vi "GUI_ENABLE_ctr (SubVI).vi"(8 "error out 2":errorcluster, 10 "Array":refnum<vi>[](array[refnum]), 11 "Visible":bool) -> (0 "error out":errorcluster)   [LabVIEW 2017]
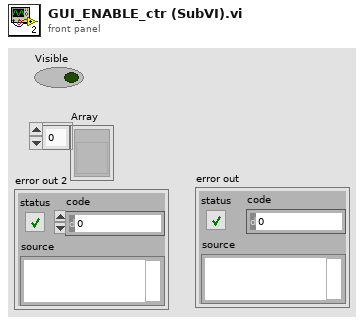
[diagram p1: front panel]
types:
  T1 = enum8{"Enabled", "Disabled", "Disabled and Grayed Out"}
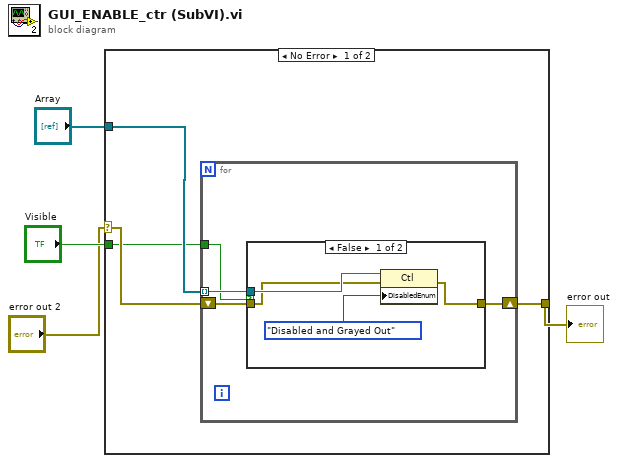
[diagram p0: block diagram]
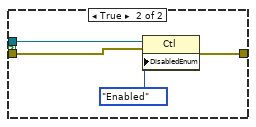
[diagram p2: hidden frame]
diagram:
  n1 = case shown="No Error" "error out 2" {
    selector: "error out 2" -> [w6 w21]
    tunnel: "Visible" -> [w5 _]
    tunnel: "Array" -> [w8 _]
    tunnel: [w7 w21] -> w2
    frame No Error {
      n2 = for {
        tunnel: w8 -> [w12] mode=indexing
        shift-right: [w11] -> w7
        shift-left: w6 -> [w10]
        tunnel: w5 -> [w9]
        n3 = case shown="False" w9 {
          tunnel: w12 -> [w15 w20]
          tunnel: [w13 w19] -> w11
          tunnel: w10 -> [w14 w18]
          frame False {
            n4 = property class="Ctl"(reference=w15, error in=w14, "DisabledEnum"=T1."Disabled and Grayed Out" ("Disabled")) -> (error out=w13:errorcluster)  [unwired: 1 out]
          }
          frame True {
            n5 = property class="Ctl"(reference=w20, error in=w18, "DisabledEnum"=T1."Enabled" ("Disabled")) -> (error out=w19:errorcluster)  [unwired: 1 out]
          }
        }
      }
    }
    frame Error {
    }
  }
  "error out" <- w2
